vi "氨氮启动器.vi"(11 "控制命令":enum16{"水样测试", "平行样测试", "加标回收", "停止"}(ring)) -> ()   [LabVIEW 2016, in "质控单元V2.lvlib"]
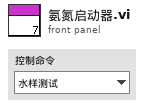
[diagram p1: front panel]
types:
  T1 = cluster{"站号":u16, "量程切换":enum32{"H", "L", "AUTO"}, "控制命令":enum16{"启动测量", "标样核查", "零点核查", "跨度核查", "空白测试", "平行样测试", "加标回收", "空白校准", "标样校准", "初始化（清洗）", "停止测试", "仪器重启", "校时", "模式设置", "测量间隔设置"}, "模式设置":enum16{"待机", "连续模式", "周期模式", "定点模式", "受控模式", "手动模式"}, "测量间隔":u16}
  T2 = cluster{"水样测试量程模式":enum16{"H", "L", "AUTO"}, "空白核查量程模式":enum16{"H", "L", "AUTO"}, "跨度核查量程模式":enum16{"H", "L", "AUTO"}, "加标回收量程模式":enum16{"H", "L", "AUTO"}}
  T3 = enum16{"启动测量", "标样核查", "零点核查", "跨度核查", "空白测试", "平行样测试", "加标回收", "空白校准", "标样校准", "初始化（清洗）", "停止测试", "仪器重启", "校时", "模式设置", "测量间隔设置"}
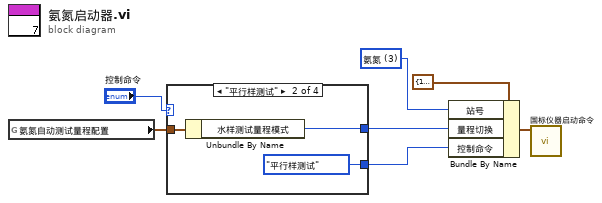
[diagram p0: block diagram]
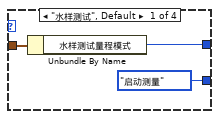
[diagram p2: hidden frame]
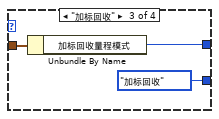
[diagram p3: hidden frame]
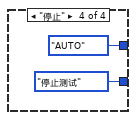
[diagram p4: hidden frame]
diagram:
  w6 = u16 3 items=["总磷"=1, "总氮"=2, "氨氮"=3, "CODMn"=21] ("站号")
  n1 = global read "系统交互.vi" "氨氮自动测试量程配置"() -> (w2:T2)
  n2 = case shown="\"平行样测试\"" "控制命令" {
    tunnel: [T3."启动测量" T3."平行样测试" T3."加标回收" T3."停止测试"] -> w3
    tunnel: w2 -> [w9 w12 w15 _]
    tunnel: [w8 w11 w14 enum16{"H", "L", "AUTO"}."AUTO" ("加标回收量程模式")] -> w1
    frame "水样测试", Default {
      n3 = Unbundle By Name(w9) -> ("水样测试量程模式"=w8:enum16{"H", "L", "AUTO"})
    }
    frame "平行样测试" {
      n4 = Unbundle By Name(w12) -> ("水样测试量程模式"=w11:enum16{"H", "L", "AUTO"})
    }
    frame "加标回收" {
      n5 = Unbundle By Name(w15) -> ("加标回收量程模式"=w14:enum16{"H", "L", "AUTO"})
    }
    frame "停止" {
    }
  }
  n6 = Bundle By Name(cluster=T1 {"站号"=1, "量程切换"=enum."AUTO", "控制命令"=enum."启动测量", "模式设置"=enum."待机", "测量间隔"=0} ("参数"), "站号"=w6, "量程切换"=w1, "控制命令"=w3) -> (w5:T1)
  n7 = call "国标仪器启动命令.vi"("参数"=w5) -> ()  [unwired: 10 in, 1 out]
